vi "Set Kinematic Parameters.vi"(8 "error in (no error)":errorcluster, 10 "kinematic parameters":T1, 11 "Finger in":refnum<class "Finger.lvclass">) -> (0 "error out":errorcluster, 3 "Finger out":refnum<class "Finger.lvclass">)   [LabVIEW 2013, in "Finger.lvclass"]
uses:
  Finger.lvclass
  controls/Kinematic Parameters.ctl
  <vilib>/Analysis/Matrix/Datatypes/RealMatrix.ctl
  <vilib>/robotics/Kinematics/Link/Joint Type.ctl
  controls/5-bar Side.ctl
  Finger.lvclass/Finger.ctl
  <vilib>/Analysis/Matrix/NI_Matrix.lvlib
  <vilib>/robotics/Kinematics/Link/NI_Robotics_Link.lvclass
panel:
  out "Parameters OK":bool
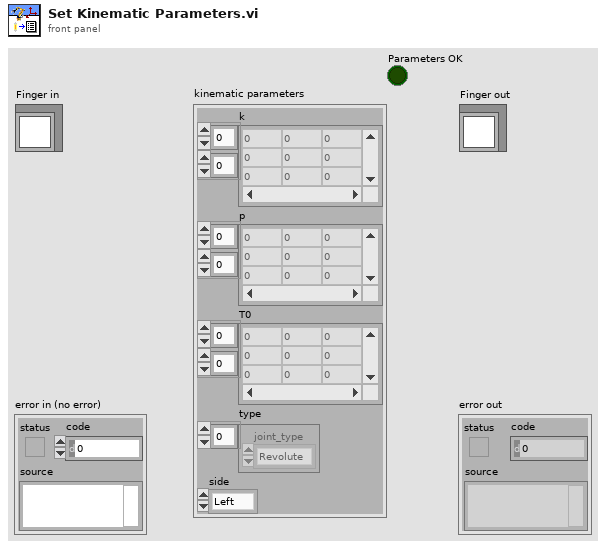
[diagram p1: front panel]
types:
  T1 = typedef "Kinematic Parameters.ctl" = cluster{"k":T2, "p":T2, "T0":T2, "type":T3[], "side":T4}
  T2 = typedef "NI_Matrix.lvlib/RealMatrix.ctl" = dbl[][]
  T3 = typedef "NI_Robotics_Link.lvclass/Joint Type.ctl" = enum16{"Revolute", "Prismatic"}
  T4 = typedef "5-bar Side.ctl" = enum16{"Left", "Right"}
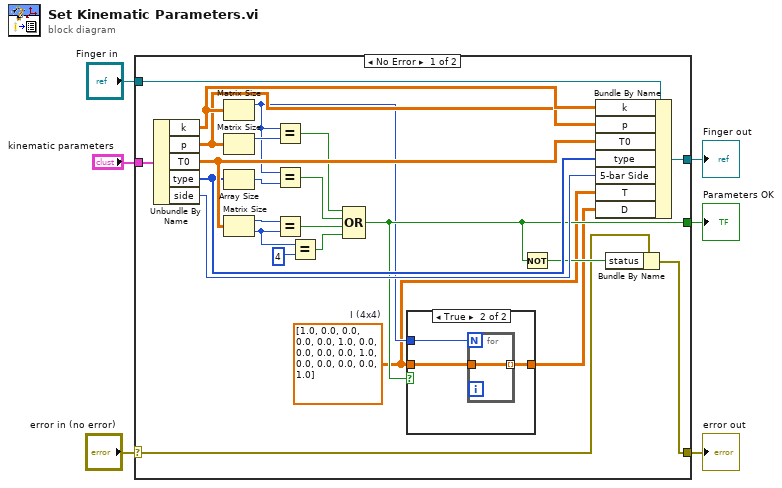
[diagram p0: block diagram]
diagram:
  n1 = case shown="No Error" "error in (no error)" {
    selector: "error in (no error)" -> [w12 w36]
    tunnel: [w11 w36] -> w5
    tunnel: [w29 w35] -> w3
    tunnel: "Finger in" -> [w30 w35]
    tunnel: "kinematic parameters" -> [w28 _]
    tunnel: [w10 _] -> w1
    frame No Error {
      w8 = T2 [[1.0, 0.0, 0.0, 0.0], [0.0, 1.0, 0.0, 0.0], [0.0, 0.0, 1.0, 0.0], [0.0, 0.0, 0.0, 1.0]]  # I (4x4)
      n2 = Unbundle By Name(w28) -> ("k"=w26:T2, "p"=w25:T2, "T0"=w23:T2, "type"=w22:T3[], "side"=w27:T4)
      n3 = Matrix Size(0:w26) -> (1:w9:i32)  [unwired: 1 out]
      n4 = Matrix Size(0:w25) -> (1:w24:i32)  [unwired: 1 out]
      n5 = Array Size(array=w22) -> (size(s)=w21:i32)
      n6 = Matrix Size(0:w23) -> (1:w20:i32, 2:w19:i32)
      n7 = Equal?(x=w9, y=w24) -> (x = y?=w17:bool)
      n8 = Equal?(x=w9, y=w21) -> (x = y?=w16:bool)
      n9 = Equal?(x=w20, y=w19) -> (x = y?=w15:bool)
      n10 = Equal?(x=w19, y=4) -> (x = y?=w14:bool)
      n11 = Compound Arithmetic op=OR(w17, w16, w15, w14) -> (w10:bool)
      n12 = case shown="True" w10 {
        tunnel: w9 -> [_ w33]
        tunnel: w8 -> [_ w31]
        tunnel: [_ w32] -> w7
        frame False {
        }
        frame True {
          n13 = for {
            N: w33 -> [_]
            tunnel: w31 -> [w34]
            tunnel: [w34] -> w32 mode=indexing
          }
        }
      }
      n14 = Not(x=w10) -> (.not. x?=w13:bool)
      n15 = Bundle By Name(cluster=w30, "k"=w26, "p"=w25, "T0"=w23, "type"=w22, "5-bar Side"=w27, "T"=w8, "D"=w7) -> (w29:refnum<class "Finger.lvclass">)
      n16 = Bundle By Name(cluster=w12, "status"=w13) -> (w11:errorcluster)
    }
    frame Error {
    }
  }
  "error out" <- w5
  "Finger out" <- w3
  "Parameters OK" <- w1
